vi "test Merge Import Routing Channels.vi"(8 "error in (no error)":errorcluster, 11 "TestCase in":refnum<class "Routing and Faulting Import Unit Tests.lvclass">) -> (0 "error out":errorcluster, 3 "TestCase out":refnum<class "Routing and Faulting Import Unit Tests.lvclass">)   [LabVIEW 2020, in "Routing and Faulting Import Unit Tests.lvclass"]
uses:
  Routing and Faulting Import Unit Tests.lvclass
  Shared/Channel States.ctl
  Shared/Routing State.ctl
  Shared/Connection.ctl
  Routing and Faulting Import Unit Tests.lvclass/Routing and Faulting Import Unit Tests.ctl
  <userlib>/_OpenG.lib/file/file.llb/Append Path to Root if Relative - Scalar__ogtk.vi
  <vilib>/addons/_JKI Toolkits/VI Tester/TestCase.llb/TestCase.lvclass
  niveristand-custom-device-testing-tools/VeriStandTestUtilities/VeriStandTestUtilities.lvlib
  <vilib>/NI VeriStand/Custom Device Tools/Custom Device Utility Library/Custom Device Utility Library.lvlib
  Scripting/Routing and Faulting Scripting.lvlib
  Shared/Routing and Faulting Shared.lvlib
  C:/Program Files (x86)/National Instruments/LabVIEW 2020/vi.lib/addons/_JKI Toolkits/VI Tester/TestCase.llb/TestCase.lvclass
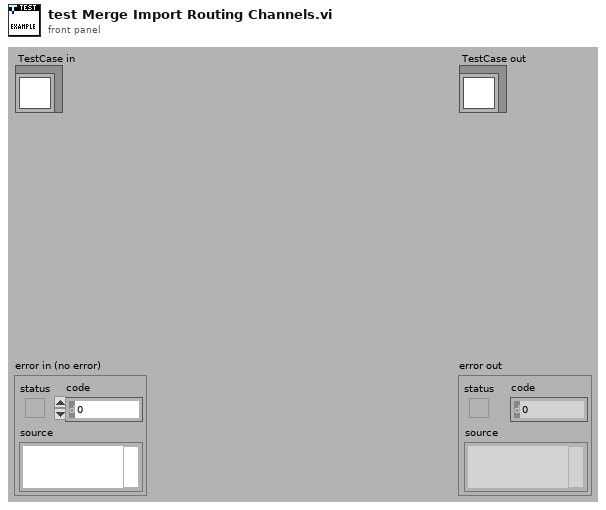
[diagram p1: front panel]
types:
  T1 = typedef "Routing and Faulting Shared.lvlib/Channel States.ctl" = T2[]
  T2 = typedef "Routing and Faulting Shared.lvlib/Routing State.ctl" = cluster{"Name":string, "Description":string, "Value":i32, "Connection List":T3[]}
  T3 = typedef "Routing and Faulting Shared.lvlib/Connection.ctl" = cluster{"Module":string, "Source":string, "Destination":string}
  T4 = cluster{"Channel Name":string, "Initial State":string, "Description":string, "State Configurations":T1}[]
  T5 = typedef "Custom Device API.lvlib/Custom Device Item Ref.ctl" = u64
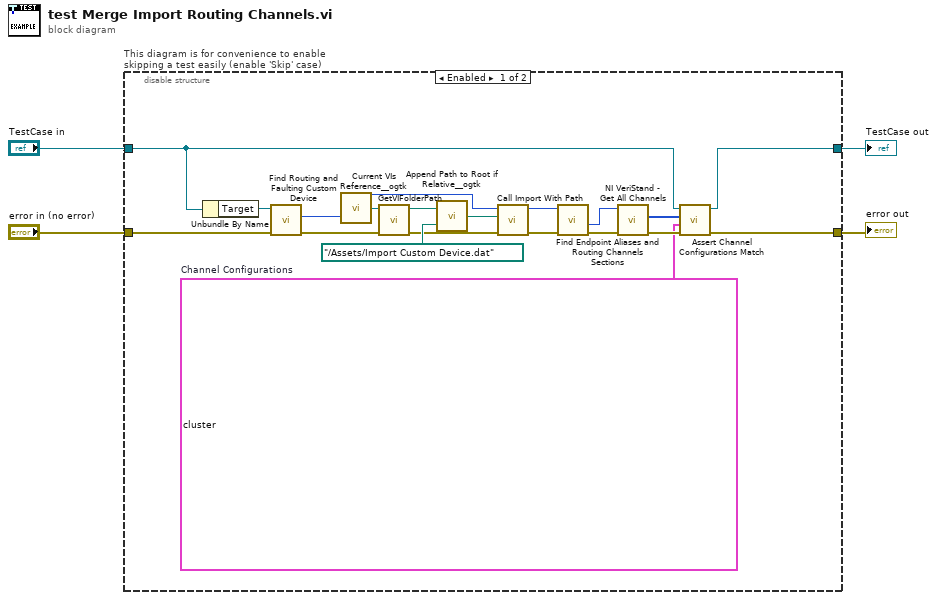
[diagram p0: block diagram]
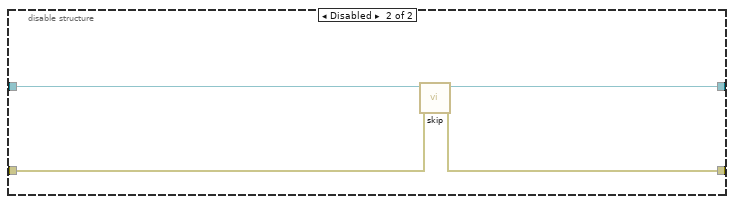
[diagram p2: hidden frame]
diagram:
  n1 = disable-structure "This diagram is for convenience to enable skipping a test easily (enable 'Skip' case)" shown="Enabled" {
    disable-tunnel: "TestCase in" -> [w11 w27]
    disable-tunnel: [w9 w25] -> w1
    disable-tunnel: [w10 w26] -> w3
    disable-tunnel: "error in (no error)" -> [w16 w24]
    frame Enabled {
      w8 = T4 [{"Channel Name"="Empty Channel", "Initial State"="No Connections", "Description"="Empty Channel", "State Configurations"=[{"Name"="No Connections", "Description"="State with no connections", "Value"=-1, "Connection List"=[]}]}, {"Channel Name"="Routing Channel", "Initial State"="One Connection", "Description"="This channel has some trivial states in it.", "State Configurations"=[{"Name"="No Connections", "Description"="State with no connections", "Value"=-1, "Connection List"=[]}, {"Name"="One Connection", "Description"="One connection in this state", "Value"=0, "Connection List"=[{"Module"="Targets/Controller/Hardware/SLSC/SLSC Chassis/Modules/Slot 2 (SLSC Switch)", "Source"="DUT_Ch0", "Destination"="LOAD_Ch0"}]}, {"Name"="Two Connections", "Description"="Two connections in this state", "Value"=10, "Connection List"=[{"Module"="Targets/Controller/Hardware/SLSC/SLSC Chassis/Modules/Slot 4 (SLSC Switch)", "Source"="DUT_Ch0", "Destination"="LOAD_Ch0"}, {"Module"="Targets/Controller/Hardware/SLSC/SLSC Chassis/Modules/Slot 2 (SLSC Switch)", "Source"="DUT_Ch0", "Destination"="LOAD_Ch0"}]}]}]  # Channel Configurations
      n2 = Unbundle By Name(w11) -> ("Target"=w14:refnum<k24>)
      n3 = call "Find Routing and Faulting Custom Device.vi"("error in"=w16, "target in"=w14) -> ("error out"=w15:errorcluster, "routing and faulting custom device"=w6:T5)  [unwired: 7 in, 1 out]
      n4 = call <userlib>:"Current VIs Reference__ogtk.vi"() -> ("Current VI's reference"=w23:refnum<vi>)  [unwired: 5 in]
      n5 = call "GetVIFolderPath.vi"("error in (no error)"=w15, "VI Reference in"=w23) -> ("error out"=w20:errorcluster, "VI Folder Path out"=w22:path)  [unwired: 8 in]
      n6 = call-poly <userlib>:"Append Path to Root if Relative__ogtk.vi"("Absolute or Relative Path"=path "../Assets/Import Custom Device.dat", "Root Path"=w22) -> ("Absolute or Appended Path"=w7:path)
      n7 = call "Call Import With Path.vi"("error in (no error)"=w20, "Path"=w7, "Routing and Faulting Custom Device Ref in"=w6) -> ("error out"=w19:errorcluster, "Routing and Faulting Custom Device Ref out"=w5:T5)  [unwired: 7 in]
      n8 = call "Find Endpoint Aliases and Routing Channels Sections.vi"("error in"=w19, "routing and faulting custom device in"=w5) -> ("error out"=w18:errorcluster, "routing channels"=w17:T5)  [unwired: 6 in, 2 out]
      n9 = call <vilib>:"NI VeriStand - Get All Channels.vi"("error in"=w18, "Section Ref in"=w17) -> ("error out"=w13:errorcluster, "Channel Refs"=w12:T5[])  [unwired: 6 in, 2 out]
      n10 = call "Assert Channel Configurations Match.vi"("error in (no error)"=w13, "Channel Configurations"=w8, "Channel Refs"=w12, "Test Case in"=w11) -> ("error out"=w10:errorcluster, "Test Case out"=w9:refnum<class "Routing and Faulting Import Unit Tests.lvclass">)  [unwired: 6 in]
    }
    frame Disabled {
      # "skip test result while test is under development"
      n11 = call <vilib>:"skip.vi"("error in (no error)"=w24, "TestCase in"=w27) -> ("error out"=w26:errorcluster, "TestCase out"=w25:refnum<class "Routing and Faulting Import Unit Tests.lvclass">)  [unwired: 8 in]
    }
  }
  "error out" <- w3
  "TestCase out" <- w1
